vi "Posiciones_Alrededor_Mina.vi"(1 "Numero_Columnas":dbl, 2 "Numero_Filas":dbl, 3 "Posicion":string) -> (0 "Posiciones_Alrededor_Mina":string[](array[string]))   [LabVIEW 2019]
doc: "Parametros -------------------------------------\n\n'Posicion_Mina': Corresponde a una cadena de texto con la posición 'x,y' de la mina en el tablero.\n'Num_Filas': Corresponde al número de filas del tablero.\n'Num_Columnas': Corresponde al número de columnas del tablero.\n\nRetorna ----------------------------------------\n\n'Posiciones_Alrededor__Mina': lista con todas las posiciones 'x,y' que se encuentran al rededor de la posición de la mina."
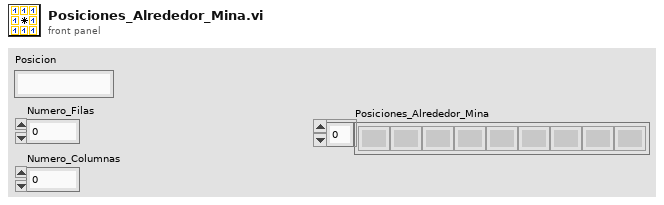
[diagram p1: front panel]
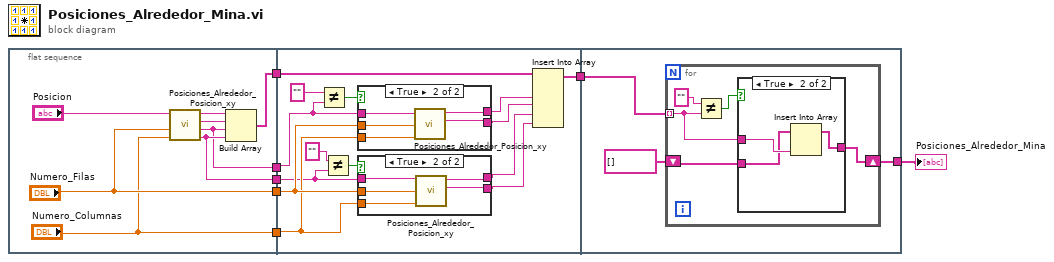
[diagram p0: block diagram]
diagram:
  n1 = flat-sequence {
    tunnel: ["Numero_Filas"] -> w6
    tunnel: ["Numero_Columnas"] -> w5
    tunnel: [w10] -> w4
    tunnel: [w9] -> w3
    tunnel: [w8] -> w2
    tunnel: w6 -> [w29]
    tunnel: w5 -> [w28]
    tunnel: w4 -> [w22]
    tunnel: w3 -> [w25]
    tunnel: w2 -> [w21]
    tunnel: [w16] -> w1
    tunnel: [w42] -> w7
    tunnel: w1 -> [w43]
    frame #0 {
      n2 = call "Posiciones_Alrededor_Posicion_xy.vi"("Num_Columnas"="Numero_Columnas", "Num_Filas"="Numero_Filas", "Posicion_Mina"="Posicion") -> ("Posicion_Derecha"=w10:string, "Posicion_Izquierda"=w9:string, "Posicion_Inferior"=w13:string, "Posicion_Superior"=w14:string)  [unwired: 1 in]
      n3 = Build Array(w14, w13, w9, w10) -> (w8:string[])
    }
    frame #1 {
      n4 = Not Equal?(x="", y=w25) -> (x != y?=w27:bool)
      n5 = Not Equal?(x="", y=w22) -> (x != y?=w23:bool)
      n6 = case shown="True" w27 {
        tunnel: w25 -> [w36 w41]
        tunnel: [w36 w38] -> w20
        tunnel: [w36 w37] -> w19
        tunnel: w29 -> [_ w40]
        tunnel: w28 -> [_ w39]
        frame False {
        }
        frame True {
          n7 = call "Posiciones_Alrededor_Posicion_xy.vi"("Num_Columnas"=w39, "Num_Filas"=w40, "Posicion_Mina"=w41) -> ("Posicion_Inferior"=w37:string, "Posicion_Superior"=w38:string)  [unwired: 1 in, 2 out]
        }
      }
      n8 = case shown="True" w23 {
        tunnel: w22 -> [w30 w35]
        tunnel: [w30 w32] -> w18
        tunnel: [w30 w31] -> w17
        tunnel: w29 -> [_ w34]
        tunnel: w28 -> [_ w33]
        frame False {
        }
        frame True {
          n9 = call "Posiciones_Alrededor_Posicion_xy.vi"("Num_Columnas"=w33, "Num_Filas"=w34, "Posicion_Mina"=w35) -> ("Posicion_Inferior"=w31:string, "Posicion_Superior"=w32:string)  [unwired: 1 in, 2 out]
        }
      }
      n10 = Insert Into Array(array=w21, new element #1=w20, new element #2=w19, new element #3=w18, new element #4=w17) -> (w16:string[])  [unwired: 1 in]
    }
    frame #2 {
      n11 = for {
        tunnel: w43 -> [w47] mode=indexing
        shift-right: [w46] -> w42
        shift-left: string[] [] -> [w45]
        n12 = Not Equal?(x="", y=w47) -> (x != y?=w48:bool)
        n13 = case shown="True" w48 {
          tunnel: w47 -> [_ w53]
          tunnel: [w50 w52] -> w46
          tunnel: w45 -> [w50 w51]
          frame False {
          }
          frame True {
            n14 = Insert Into Array(array=w51, new element=w53) -> (w52:string[])  [unwired: 1 in]
          }
        }
      }
    }
  }
  "Posiciones_Alrededor_Mina" <- w7
